vi "Controller Output.vi"() -> ()   [LabVIEW 2016]
uses:
  YSH_XBOX360_joystick.ctl
panel:
  out "Controller Output":T1 {"Joy1 Y-axis" scale=-32767.0..32767.0; "Joy2 Y-axis" scale=-32767.0..32767.0; "Joy2 X-axis" scale=-32767.0..32767.0; "Joy1 X-axis" scale=-32767.0..32767.0; "Z axis - LT~RT" scale=-32767.0..32767.0; "DPad" scale=0.0..360.0}
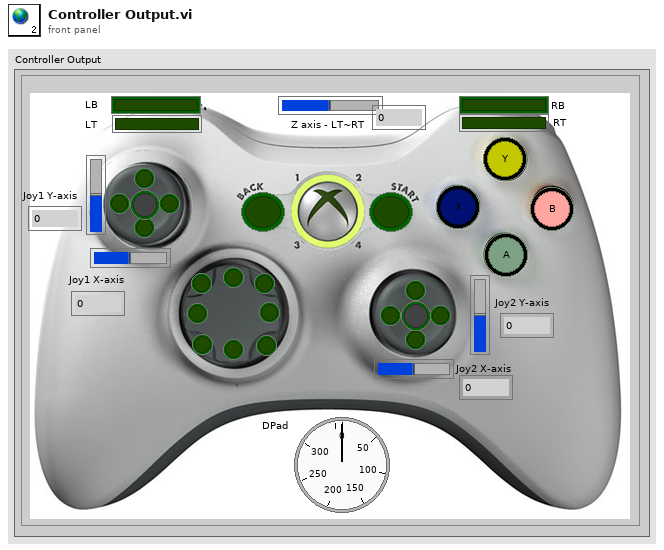
[diagram p1: front panel]
types:
  T1 = typedef "YSH_XBOX360_joystick.ctl" = cluster{"RR":bool, "RL":bool, "RD":bool, "RU":bool, "LR":bool, "LL":bool, "LD":bool, "LU":bool, "Back":bool, "Start":bool, "DPad":dbl, "D Pad":cluster{"0":bool, "45":bool, "90":bool, "135":bool, "180":bool, "215":bool, "270":bool, "315":bool}, "A":bool, "B":bool, "X":bool, "Y":bool, "LB":bool, "RB":bool, "LT":bool, "RT":bool, "Left Joy Push":bool, "Right Joy Push":bool, "Z axis - LT~RT":i32, "Joy1 X-axis":i32, "Joy2 X-axis":i32, "Joy2 Y-axis":i32, "Joy1 Y-axis":i32}
diagram:
